vi "gearValue.vi"() -> ()   [LabVIEW 2016]
panel:
  out "gearValue":dbl
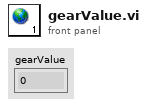
[diagram p1: front panel]
diagram:
